vi "Configure Noise.vi"(8 "error in (no error)":errorcluster, 9 "Noise Level (0%)":dbl, 10 "Enable Noise (F: Disable)":bool, 11 "VISA resource name":refnum<visa-resource-name>) -> (0 "error out":errorcluster, 3 "VISA resource name out":refnum<visa-resource-name>)   [LabVIEW 2016, in "Tektronix DPO MSO 2000 4000 Series.lvlib"]
doc: "Configures the Arbitrary Function Generator additive noise.\n\n<B>Notes:</B>\n(1) This VI is available for MDO3000 Series only.\n\n(2) Requires the MDO3AFG option to be installed."
uses:
  Tektronix DPO MSO 2000 4000 Series.lvlib
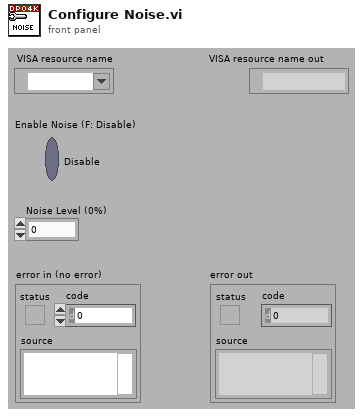
[diagram p1: front panel]
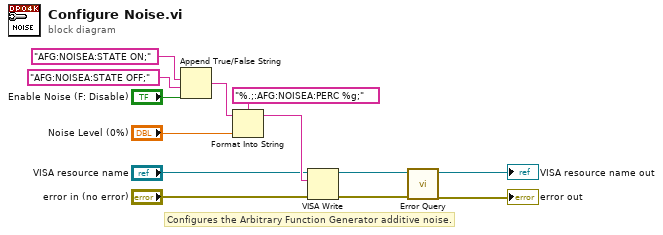
[diagram p0: block diagram]
diagram:
  # "Configures the Arbitrary Function Generator additive noise."
  n1 = Append True/False String(1:"Enable Noise (F: Disable)", 2:"AFG:NOISEA:STATE OFF;", 3:"AFG:NOISEA:STATE ON;") -> (0:w10:string)  [unwired: 1 in]
  n2 = Format Into String(format string="%.;:AFG:NOISEA:PERC %g;", initial string=w10, "Noise Level (0%)") -> (resulting string=w7:string)  [unwired: 1 in, 1 out]
  n3 = VISA Write(VISA resource name="VISA resource name", write buffer=w7, error in (no error)="error in (no error)") -> (VISA resource name out=w5:refnum<visa-resource-name>, error out=w4:errorcluster)  [unwired: 1 out]
  n4 = call "Error Query.vi"("error in (no error)"=w4, "VISA resource name"=w5) -> ("error out"=→"error out":errorcluster, "VISA resource name out"=→"VISA resource name out":refnum<visa-resource-name>)  [unwired: 6 in, 2 out]
